vi "Hardware-UEGO-Host.vi"() -> ()   [LabVIEW 2016]
panel:
  out "UEGO2Hot":bool
  out "UEGO2Temp":sgl
  out "UEGO1Hot":bool
  out "UEGO1Temp":sgl
  out "UEGODiagnostics":sgl[](array[numeric])
  out "UEGOSensorResults":sgl[](array[numeric])
  out "_UEGO Diagnostics":T1={"UEGO1HeaterFault"=192, "UEGO1SensorFault"=63, "UEGO2HeaterFault"=192, "UEGO2SensorFault"=63, "UEGOFuseStatus"=0, "Battery (V)"=0.0, "LSUType"=0} caption="UEGO Diagnostics" {"LSUType" items=["LSU 4.9", "LSU 4.2"]; "UEGOFuseStatus" items=["FUSE OK", "FUSE BLOWN"]; "UEGO2SensorFault" items=["NO FAULT"=63, "SHORT TO GND OR BATT"=0]; "UEGO2HeaterFault" items=["SHORT TO GROUND"=0, "OPEN CIRCUIT"=64, "SHORT TO BATTERY"=128, "NO FAULT"=192]; "UEGO1SensorFault" items=["NO FAULT"=63, "SHORT TO GND OR BATT"=0]; "UEGO1HeaterFault" items=["SHORT TO GROUND"=0, "OPEN CIRCUIT"=64, "SHORT TO BATTERY"=128, "NO FAULT"=192]}
  out "_UEGO Sensor Results":T2 caption="UEGO Sensor Results"
  in  "UEGO2Range":bool
  in  "UEGO1Enable":bool
  in  "UEGO2Enable":bool
  in  "UEGO1Range":bool
  in  "UEGOFilterCutOff":sgl=10.0
  # "UEGO Diagnostics"
  # "UEGO Sensor Results"
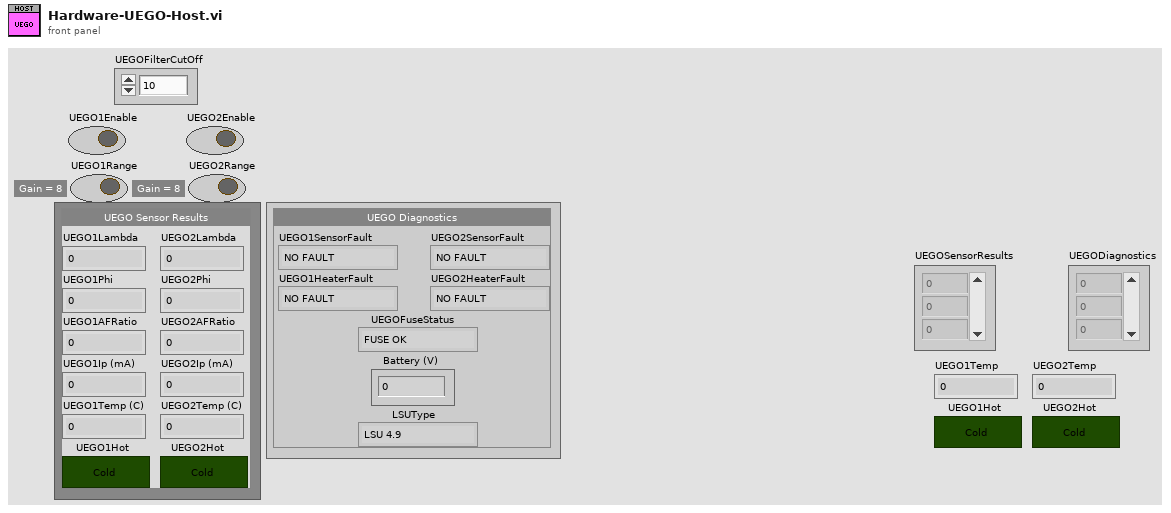
[diagram p1: front panel]
types:
  T1 = cluster{"UEGO1HeaterFault":u8, "UEGO1SensorFault":u8, "UEGO2HeaterFault":u8, "UEGO2SensorFault":u8, "UEGOFuseStatus":u8, "Battery (V)":sgl, "LSUType":u8}
  T2 = cluster{"UEGO1Lambda":sgl, "UEGO1Phi":sgl, "UEGO1AFRatio":sgl, "UEGO2Lambda":sgl, "UEGO2AFRatio":sgl, "UEGO2Phi":sgl, "UEGO1Ip (mA)":sgl, "UEGO2Ip (mA)":sgl, "UEGO1Temp (C)":sgl, "UEGO1Hot":bool, "UEGO2Temp (C)":sgl, "UEGO2Hot":bool}
  T3 = cluster{"UEGODiagnostics[0]":sgl, "UEGODiagnostics[1]":sgl, "UEGODiagnostics[2]":sgl, "UEGODiagnostics[3]":sgl, "UEGODiagnostics[4]":sgl, "UEGODiagnostics[5]":sgl, "UEGODiagnostics[6]":sgl}
  T4 = cluster{"Numeric":sgl, "Numeric":sgl, "Numeric":sgl, "Numeric":sgl, "Numeric":sgl, "Numeric":sgl, "Numeric":sgl, "Numeric":sgl, "UEGO1Temp":sgl, "UEGO1Hot":bool, "UEGO2Temp":sgl, "UEGO2Hot":bool}
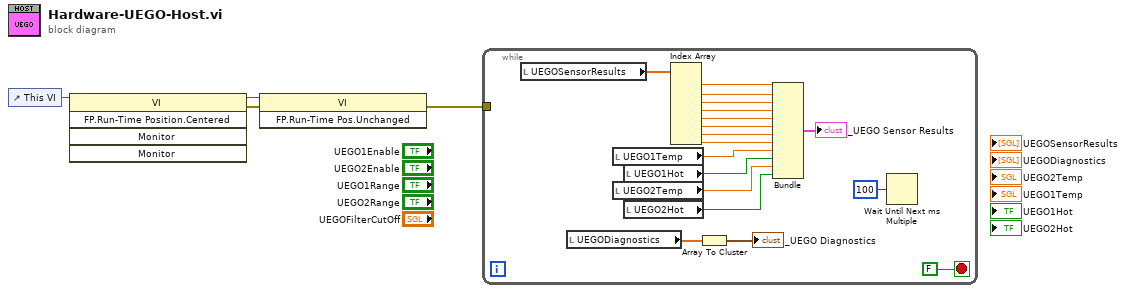
[diagram p0: block diagram]
diagram:
  n1 = control-ref of="This VI"() -> (w4:refnum<vi>)
  n2 = invoke class="VI" method="FP.Run-Time Position.Centered"(reference=w4) -> (reference out=w3:refnum<vi>, error out=w2:errorcluster)  [unwired: 4 in, 3 out]
  n3 = invoke class="VI" method="FP.Run-Time Pos.Unchanged"(reference=w3, error in=w2) -> (error out=w1:errorcluster)  [unwired: 1 in, 2 out]
  n4 = while {
    tunnel: w1 -> [_]
    stop <- FALSE stop-if-true
    n5 = local read "UEGOSensorResults"() -> (w12:sgl[])
    n6 = local read "UEGODiagnostics"() -> (w21:sgl[])
    n7 = local read "UEGO1Temp"() -> (w11:sgl)
    n8 = local read "UEGO2Temp"() -> (w8:sgl)
    n9 = local read "UEGO1Hot"() -> (w7:bool)
    n10 = local read "UEGO2Hot"() -> (w9:bool)
    n11 = Index Array(array=w12) -> (element #1=w13:sgl, element #2=w14:sgl, element #3=w15:sgl, element #4=w16:sgl, element #5=w17:sgl, element #6=w18:sgl, element #7=w19:sgl, element #8=w20:sgl)  [unwired: 8 in]
    n12 = Array To Cluster(array=w21) -> (cluster=→"_UEGO Diagnostics":T3)
    n13 = Bundle("Numeric"=w13, "Numeric"=w14, "Numeric"=w15, "Numeric"=w16, "Numeric"=w17, "Numeric"=w18, "Numeric"=w19, "Numeric"=w20, "UEGO1Temp"=w11, "UEGO1Hot"=w7, "UEGO2Temp"=w8, "UEGO2Hot"=w9) -> (→"_UEGO Sensor Results":T4)  [unwired: 1 in]
    n14 = Wait Until Next ms Multiple(millisecond multiple=u32 100) -> ()  [unwired: 1 out]
  }
